vi "Read Power Settings.vi"(8 "error in (no error)":errorcluster, 11 "Parttype":refnum<vi>) -> (0 "error out":errorcluster, 2 "ECU Info":string[](array[string]), 3 "Power setting":string[](array[string]))   [LabVIEW 2014]
uses:
  typedefs/parttype.ctl
  <vilib>/Utility/config.llb/Read Key (String).vi
  <vilib>/Utility/config.llb/NI_LVConfig.lvlib
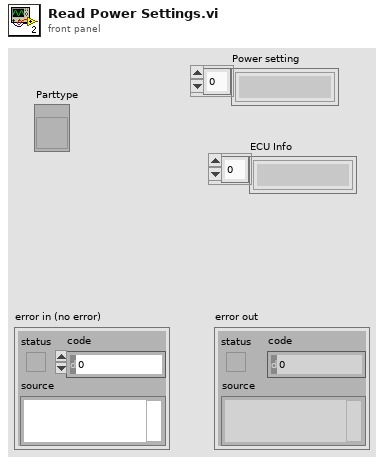
[diagram p1: front panel]
types:
  T1 = typedef "NI_LVConfig.lvlib/Config Data RefNum.ctl" = refnum<k1>
  T2 = typedef "parttype.ctl" = enum16{"NMS", "B-SUV"}
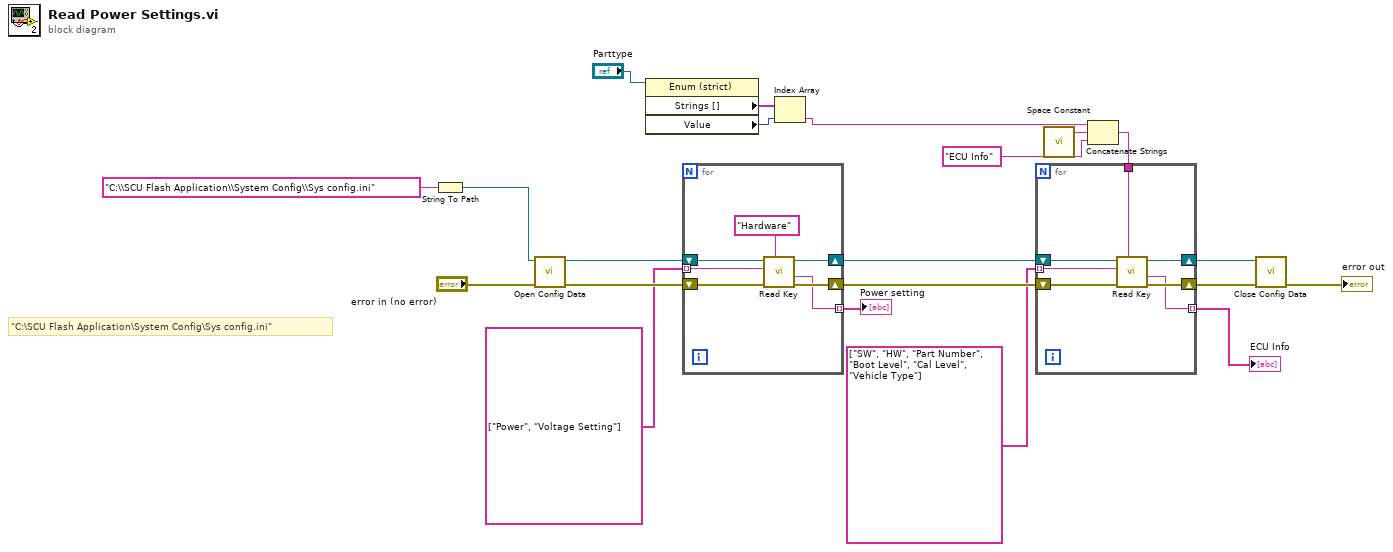
[diagram p0: block diagram]
diagram:
  # "\"C:\\SCU Flash Application\\System Config\\Sys config.ini\""
  n1 = String To Path(string="C:\\SCU Flash Application\\System Config\\Sys config.ini" ("name or relative path")) -> (path=w9:path)
  n2 = call <vilib>:"Open Config Data.vi"("error in (no error)"="error in (no error)", "configuration file path"=w9) -> ("error out"=w20:errorcluster, "refnum"=w21:T1)  [unwired: 7 in, 1 out]
  n3 = property class="Enum (strict)"(reference="Parttype") -> ("Strings []"=w6:string[], "Value"=w7:T2)  [unwired: 1 in, 2 out]
  n4 = for {
    tunnel: string[] ["Power", "Voltage Setting"] -> [w25] mode=indexing
    shift-right: [w24] -> w14
    shift-left: w21 -> [w28]
    shift-right: [w23] -> w15
    shift-left: w20 -> [w27]
    tunnel: [w22] -> w16 mode=indexing
    n5 = call-poly <vilib>:"Read Key.vi"("section"="Hardware", "error in (no error)"=w27, "key"=w25, "refnum"=w28) -> ("error out"=w23:errorcluster, "value"=w22:string, "refnum out"=w24:T1)  [unwired: 4 in, 1 out]
  }
  "Power setting" <- w16
  n6 = Index Array(array=w6, index=w7) -> (element=w4:string)
  n7 = call <vilib>:"Space Constant.vi"() -> ("String"=w3:string)
  n8 = Concatenate Strings(w4, w3, "ECU Info" ("section")) -> (w1:string)
  n9 = for {
    tunnel: string[] ["SW", "HW", "Part Number", "Boot Level", "Cal Level", "Vehicle Type"] -> [w33] mode=indexing
    shift-right: [w32] -> w11
    shift-left: w14 -> [w35]
    shift-right: [w31] -> w12
    shift-left: w15 -> [w34]
    tunnel: [w30] -> w10 mode=indexing
    tunnel: w1 -> [w29]
    n10 = call-poly <vilib>:"Read Key.vi"("section"=w29, "error in (no error)"=w34, "key"=w33, "refnum"=w35) -> ("error out"=w31:errorcluster, "value"=w30:string, "refnum out"=w32:T1)  [unwired: 4 in, 1 out]
  }
  "ECU Info" <- w10
  n11 = call <vilib>:"Close Config Data.vi"("error in (no error)"=w12, "refnum"=w11) -> ("error out"=→"error out":errorcluster)  [unwired: 8 in, 1 out]
